vi "加标回收数据插入.vi"(8 "error in (no error)":errorcluster, 11 "data in":T1={"时间"=timestamp(0 s since 1904-01-01), "参数"="", "数据类型"="N", "加标回收率"=0.0, "加标前水样测试时间"=timestamp(0 s since 1904-01-01), "加标前水样浓度值"=0.0, "加标后水样浓度值"=0.0, "加标母液浓度值"=0.0, "加标体积"=0.0, "加标水杯定容体积"=0.0}) -> (0 "error out":errorcluster)   [LabVIEW 2016, in "质控单元V2.lvlib"]
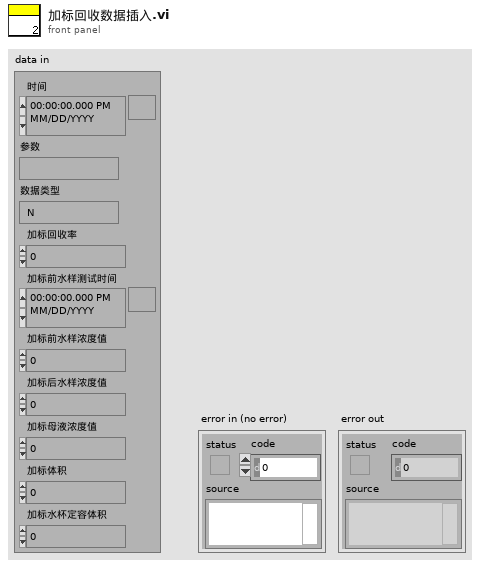
[diagram p1: front panel]
types:
  T1 = cluster{"时间":timestamp, "参数":string, "数据类型":string, "加标回收率":sgl, "加标前水样测试时间":timestamp, "加标前水样浓度值":sgl, "加标后水样浓度值":sgl, "加标母液浓度值":sgl, "加标体积":sgl, "加标水杯定容体积":sgl}
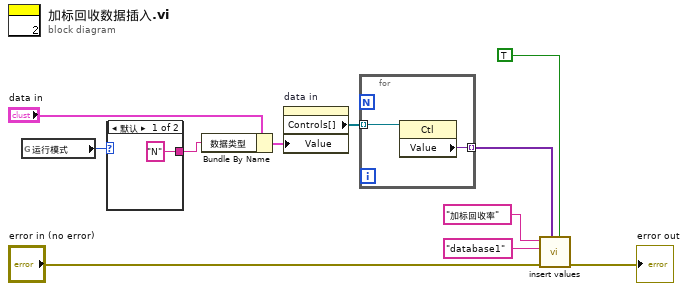
[diagram p0: block diagram]
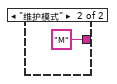
[diagram p2: hidden frame]
diagram:
  n1 = global read "系统交互.vi" "运行模式"() -> (w8:enum16{"维护模式", "常规模式", "应急模式", "质控模式"})
  n2 = case shown="默认" w8 {
    tunnel: ["N" "M"] -> w7
    frame Default {
    }
    frame "维护模式" {
    }
  }
  n3 = Bundle By Name(cluster="data in", "数据类型"=w7) -> (w9:T1)
  n4 = property on="data in" class="Clust (严格)"("Value"=w9) -> ("Controls[]"=w11:refnum<vi>[])  [unwired: 2 in, 2 out]
  n5 = for {
    tunnel: w11 -> [w15] mode=indexing
    tunnel: [w14] -> w2 mode=indexing
    n6 = property class="Ctl"(reference=w15) -> ("Value"=w14:variant)  [unwired: 1 in, 2 out]
  }
  n7 = call "insert values.vi"("是否创建唯一键"=TRUE, "data"=w2, "错误输入（无错误）"="error in (no error)", "database"="database1", "Tabe Name"="加标回收率" ("table")) -> ("错误输出"=→"error out":errorcluster)  [unwired: 6 in]
